vi "Set Remove SourceOnly Tag for VI in Memory.vi"(8 "error in":errorcluster, 10 "VI Ref in":refnum<vi>, 11 "Set":bool) -> (0 "error out":errorcluster, 1 "Lock State":T1(ring), 2 "VI Ref out":refnum<vi>)   [LabVIEW 2020]
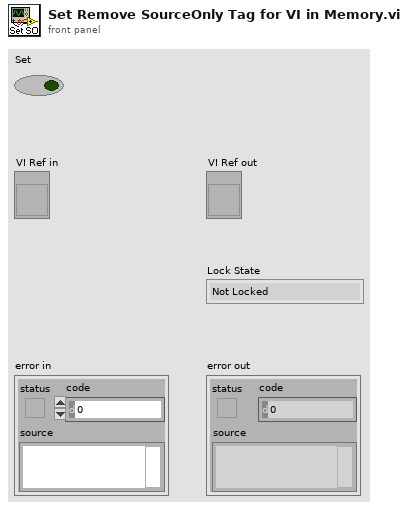
[diagram p1: front panel]
types:
  T1 = enum32{"Not Locked", "Invalid Password", "Locked (No Password)"}
  T2 = enum32{"invalid lock state", "Not Locked", "Locked (No Password)", "Password-protected"}
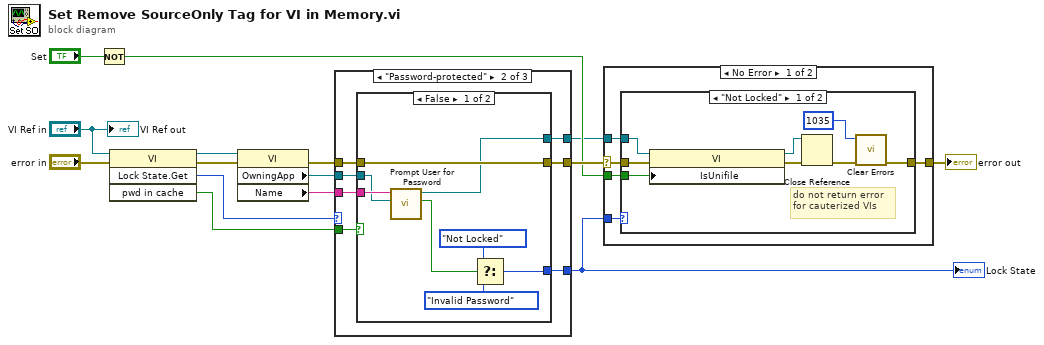
[diagram p0: block diagram]
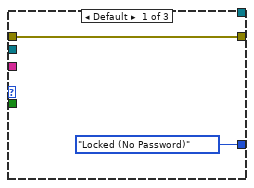
[diagram p4: hidden frame]
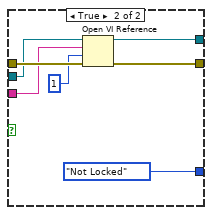
[diagram p5: hidden frame]
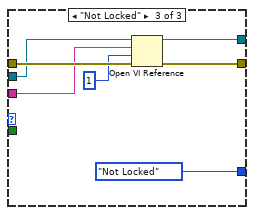
[diagram p6: hidden frame]
diagram:
  n1 = Not(x="Set") -> (.not. x?=w9:bool)
  n2 = invoke class="VI" method="Lock State.Get"(reference="VI Ref in", error in="error in") -> (reference out=w6:refnum<vi>, error out=w13:errorcluster, "Get Lock State"=w8:T2, "pwd in cache"=w7:bool)  [unwired: 2 in]
  n3 = property class="VI"(reference=w6, error in=w13) -> (error out=w12:errorcluster, "OwningApp"=w2:refnum<vi>, "Name"=w3:string)  [unwired: 1 out]
  n4 = case shown="\"Password-protected\"" w8 {
    tunnel: [T1."Locked (No Password)" ("Lock State") w21 T1."Not Locked" ("Lock State")] -> w5
    tunnel: w7 -> [_ w22 _]
    tunnel: w3 -> [_ w20 w44]
    tunnel: w12 -> [w17 w24 w46]
    tunnel: [w17 w23 w45] -> w11
    tunnel: [_ w19 w41] -> w4
    tunnel: w2 -> [_ w18 w40]
    frame Default {
    }
    frame "Password-protected" {
      n5 = case shown="False" w22 {
        tunnel: [w26 T1."Not Locked" ("Lock State")] -> w21
        tunnel: w20 -> [w31 w35]
        tunnel: [w30 w34] -> w19
        tunnel: w24 -> [w32 w39]
        tunnel: [w32 w38] -> w23
        tunnel: w18 -> [w25 w33]
        frame False {
          n6 = call <vilib>:"Prompt User for Password.vi"("reference"=w25, "VI Name"=w31) -> ("Password Valid?"=w29:bool, "VI Ref Out"=w30:refnum<vi>)  [unwired: 8 in]
          n7 = Select(t=T1."Not Locked" ("Lock State"), s=w29, f=T1."Invalid Password" ("Lock State")) -> (s? t:f=w26:T1)
        }
        frame True {
          n8 = Open VI Reference(application reference (local)=w33, vi path=w35, options=1, error in (no error)=w39) -> (vi reference=w34:refnum<vi>, error out=w38:errorcluster)  [unwired: 2 in]
        }
      }
    }
    frame "Not Locked" {
      n9 = Open VI Reference(application reference (local)=w40, vi path=w44, options=1, error in (no error)=w46) -> (vi reference=w41:refnum<vi>, error out=w45:errorcluster)  [unwired: 2 in]
    }
  }
  "Lock State" <- w5
  n10 = case shown="No Error" w11 {
    selector: w11 -> [w50 w61]
    tunnel: [w51 w61] -> w15
    tunnel: w9 -> [w49 _]
    tunnel: w5 -> [w48 _]
    tunnel: w4 -> [w47 _]
    frame No Error {
      n11 = case shown="\"Not Locked\"" w48 {
        tunnel: [w56 w60] -> w51
        tunnel: w49 -> [w55 _]
        tunnel: w47 -> [w54 _]
        tunnel: w50 -> [w58 w60]
        frame "Not Locked" {
          # "do not return error\nfor cauterized VIs"
          n12 = property class="VI"(reference=w54, error in=w58, "IsUnifile"=w55) -> (reference out=w53:refnum<vi>, error out=w59:errorcluster)
          n13 = Close Reference(reference=w53, error in (no error)=w59) -> (error out=w57:errorcluster)
          n14 = call <vilib>:"Clear Errors.vi"("error in (no error)"=w57, "specific error code to clear (0: all)"=1035 ("y")) -> ("error out"=w56:errorcluster)  [unwired: 4 in, 1 out]
        }
        frame Default {
        }
      }
    }
    frame Error {
    }
  }
  "error out" <- w15
  "VI Ref out" <- "VI Ref in"
